vi "Start Collimation.vi"(0 "Motion Controller in":refnum<class "Motion Controller.lvclass">, 5 "Beam Profiler in":refnum<class "Beam Profiler.lvclass">, 7 "Start position":dbl[unit], 11 "error in (no error)":errorcluster) -> (2 "Cancel Test":bool, 4 "Motion Controller out":refnum<class "Motion Controller.lvclass">, 6 "Beam Profiler out":refnum<class "Beam Profiler.lvclass">, 8 "Peak responsivity [%,0-100]":dbl, 10 "Knife Edge":T1={"X"=nan, "Y"=nan}, 14 "Stop position":dbl[unit]=0.015, 15 "error out":errorcluster caption="错误输出")   [LabVIEW 2018]
uses:
  <instrlib>/nLight Instruments/Motion Controller/Motion Controller.lvclass
  <instrlib>/nLight Instruments/Beam Profiler/Beam profiler XY distance value pair.ctl
  <instrlib>/nLight Instruments/Beam Profiler/Beam Profiler.lvclass
  <instrlib>/nLight Instruments/Motion Controller/Axis index.ctl
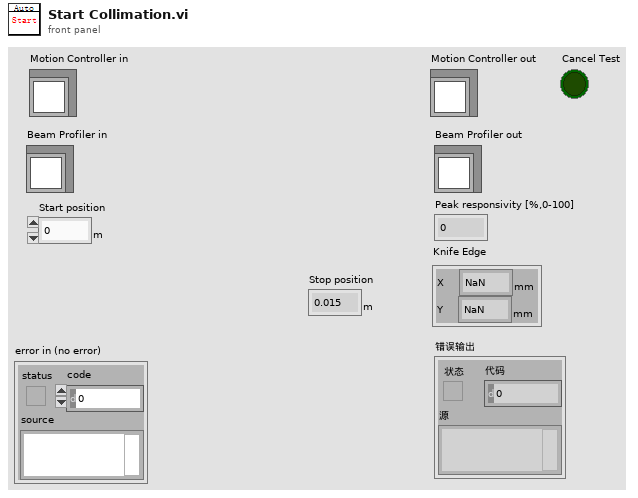
[diagram p1: front panel]
types:
  T1 = typedef "Beam Profiler.lvclass/Beam profiler XY distance value pair.ctl" = cluster{"X":dbl[unit], "Y":dbl[unit]}
  T2 = typedef "Motion Controller.lvclass/Axis index.ctl" = i32
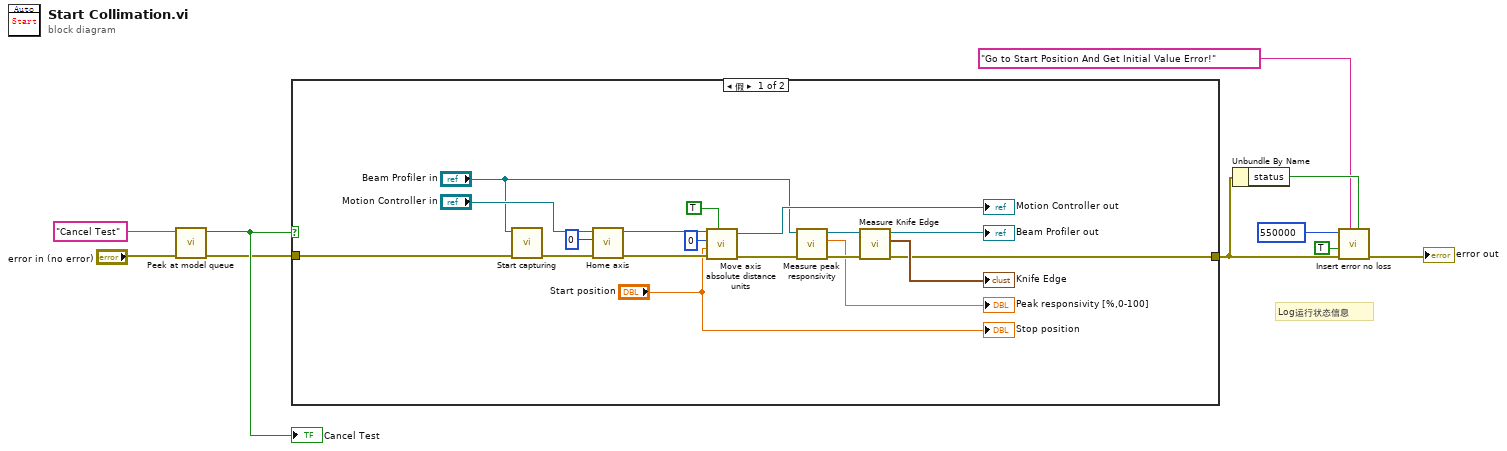
[diagram p0: block diagram]
diagram:
  # "Log运行状态信息"
  n1 = call "Peek at model queue.vi"("error in (no error)"="error in (no error)", "Check for specific pending state (don't check)"="Cancel Test") -> ("error out"=w7:errorcluster, "Specific pending state found"=w9:bool)  [unwired: 6 in, 2 out]
  "Cancel Test" <- w9
  n2 = case shown="假" w9 {
    tunnel: w7 -> [w17 w29]
    tunnel: [w16 w29] -> w4
    frame False {
      n3 = call-dynamic "Start capturing.vi"("error in (no error)"=w17, "Beam Profiler in"="Beam Profiler in") -> ("error out"=w18:errorcluster)  [unwired: 8 in, 1 out]
      n4 = call-dynamic "Home axis.vi"("error in (no error)"=w18, "Axis index"=T2 0, "Motion Controller in"="Motion Controller in") -> ("error out"=w15:errorcluster, "Motion Controller out"=w14:refnum<class "Motion Controller.lvclass">)  [unwired: 7 in]
      n5 = call <instrlib>:"Move axis absolute distance units.vi"("Wait? (T)"=TRUE, "error in (no error)"=w15, "Move location"="Start position", "Axis index"=T2 0, "Motion Controller in"=w14) -> ("error out"=w25:errorcluster, "Motion Controller out"=→"Motion Controller out":refnum<class "Motion Controller.lvclass">)  [unwired: 5 in]
      n6 = call-dynamic "Measure peak responsivity.vi"("error in (no error)"=w25, "Beam Profiler in"="Beam Profiler in") -> ("error out"=w24:errorcluster, "Peak responsivity [%,0-100]"=→"Peak responsivity [%,0-100]":dbl, "Beam Profiler out"=w23:refnum<class "Beam Profiler.lvclass">)  [unwired: 7 in]
      n7 = call-dynamic "Measure Knife Edge.vi"("error in (no error)"=w24, "Beam Profiler 输入"=w23) -> ("error out"=w16:errorcluster, "Knife Edge"=→"Knife Edge":T1, "Beam Profiler 输出"=→"Beam Profiler out":refnum<class "Beam Profiler.lvclass">)  [unwired: 7 in]
      "Stop position" <- "Start position"
    }
    frame True {
    }
  }
  n8 = Unbundle By Name(w4) -> ("status"=w3:bool)
  n9 = call <userlib>:"Insert error no loss.vi"("Add error? (T)"=w3, "error message"="Go to Start Position And Get Initial Value Error!" ("format string"), "error in (no error)"=w4, "Error = T, Warning = F (T)"=TRUE, "error code"=550000) -> ("error out"=→"error out":errorcluster)  [unwired: 4 in]
